vi "Configure Relays.vi"(6 "Alarm Type (0: Low Alarm)":u16(ring) items=["Low Alarm", "High Alarm", "Both Alarms"], 7 "Relay Mode (0: Off)":u16(ring) items=["Off", "On", "Alarms", "Sample Heater Zone", "Warmup Heater Zone"], 8 "error in (no error)":errorcluster, 9 "Channel (1:1)":u16(ring)=1 items=["Scan Channel", "1", "2", "3", "4", "5", "6", "7", "8", "9", "10", "11", "12", "13", "14", "15", "16", "A (Control Input)"], 10 "Relay to Configure (1: Low)":u16(ring)=1 items=["Low"=1, "High"=2], 11 "VISA resource name":refnum<visa-resource-name>) -> (0 "error out":errorcluster, 3 "VISA resource name out":refnum<visa-resource-name>)   [LabVIEW 2015, in "Lake Shore 372.lvlib"]
doc: "Configures the parameters of relay control."
uses:
  Lake Shore 372.lvlib
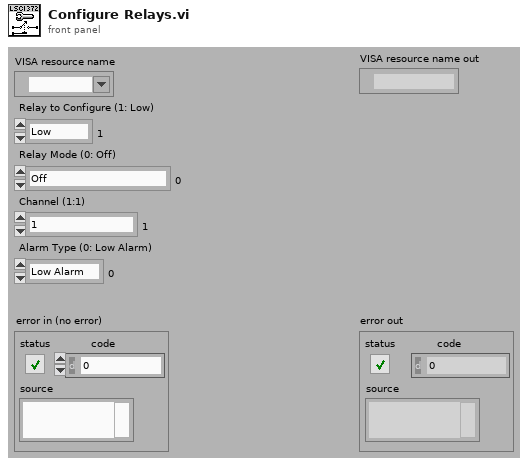
[diagram p1: front panel]
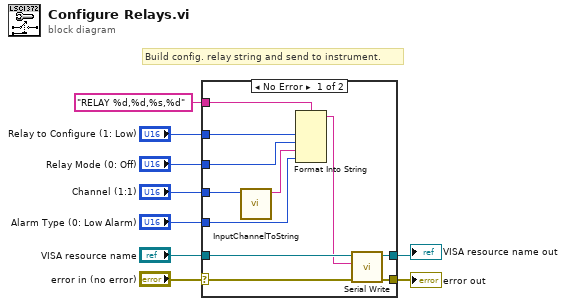
[diagram p0: block diagram]
diagram:
  # "Build config. relay string and send to instrument."
  n1 = case shown="No Error" "error in (no error)" {
    selector: "error in (no error)" -> [w12 w21]
    tunnel: "Relay to Configure (1: Low)" -> [w10 _]
    tunnel: "VISA resource name" -> [w20 w22]
    tunnel: [w19 w21] -> w7
    tunnel: [w18 w22] -> w6
    tunnel: "RELAY %d,%d,%s,%d" -> [w17 _]
    tunnel: "Relay Mode (0: Off)" -> [w16 _]
    tunnel: "Alarm Type (0: Low Alarm)" -> [w15 _]
    tunnel: "Channel (1:1)" -> [w11 _]
    frame No Error {
      n2 = call "InputChannelToString.vi"("Channel (1)"=w11) -> ("Channel Str"=w13:string)  [unwired: 10 in]
      n3 = Format Into String(format string=w17, w10, w16, w13, w15) -> (resulting string=w14:string)  [unwired: 2 in, 1 out]
      n4 = call "Serial Write.vi"("error in (no error)"=w12, "Write Buffer (\"\")"=w14, "VISA resource name"=w20) -> ("error out"=w19:errorcluster, "VISA resource name out"=w18:refnum<visa-resource-name>)  [unwired: 6 in, 1 out]
    }
    frame Error {
    }
  }
  "error out" <- w7
  "VISA resource name out" <- w6
